vi "Write Display Format.vi"(5 "Display Format":T1, 9 "NumericText in":refnum<class "NumericText.lvclass">) -> (3 "NumericText out":refnum<class "NumericText.lvclass">)   [LabVIEW 2014, in "NumericText.lvclass"]
uses:
  NumericText.lvclass
  <vilib>/Utility/miscctls.llb/LVFormatAndPrecisionTypeDef.ctl
  NumericText.lvclass/NumericText.ctl
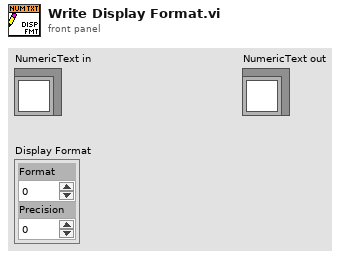
[diagram p1: front panel]
types:
  T1 = typedef "LVFormatAndPrecisionTypeDef.ctl" = cluster{"Format":u8, "Precision":u8}
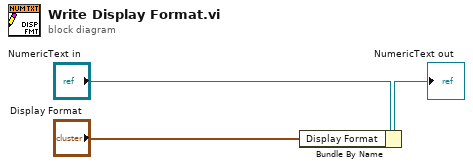
[diagram p0: block diagram]
diagram:
  n1 = Bundle By Name(cluster="NumericText in", "Display Format"="Display Format") -> (→"NumericText out":refnum<class "NumericText.lvclass">)
